vi "Send.vi"(8 "error in (no error)":errorcluster, 10 "Message":refnum<class "BaseMessage.lvclass">, 11 "MultiReader in":refnum<class "MultiReader.lvclass">) -> (0 "error out":errorcluster, 2 "Sent Message":refnum<class "BaseMessage.lvclass">, 3 "MultiReader out":refnum<class "MultiReader.lvclass">)   [LabVIEW 2018, in "MultiReader.lvclass"]
doc: "Send a message to the remote destination"
uses:
  MultiReader.lvclass
  Message/BaseMessage/BaseMessage.lvclass
  MultiReader.lvclass/MultiReader.ctl
  BaseReader/BaseReader.lvclass
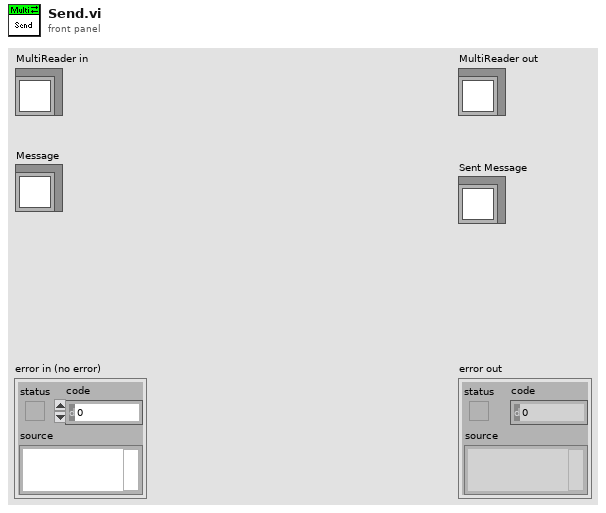
[diagram p1: front panel]
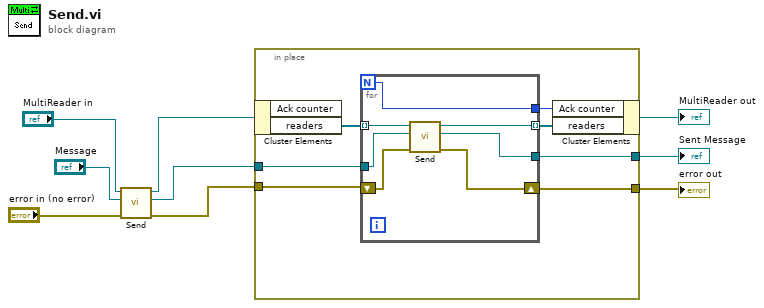
[diagram p0: block diagram]
diagram:
  n1 = call-parent "Send.vi"("error in (no error)"="error in (no error)", "Message"="Message", "BaseReader in"="MultiReader in") -> ("error out"=w4:errorcluster, "Sent Message"=w2:refnum<class "BaseMessage.lvclass">, "BaseReader out"=w6:refnum<class "MultiReader.lvclass">)  [unwired: 6 in]
  n2 = in-place {
    in-place-border: w4 -> [w14]
    in-place-border: [w13] -> w3
    in-place-border: w2 -> [w12]
    in-place-border: [w11] -> w1
    n3 = in-place-cluster #1(w6) -> ("readers"=w16:refnum<class "BaseReader.lvclass">[])  [unwired: 1 out]
    n4 = for {
      N -> [w17]
      tunnel: w16 -> [w23] mode=indexing
      tunnel: [w22] -> w15 mode=indexing
      shift-right: [w19] -> w13
      shift-left: w14 -> [w20]
      tunnel: w12 -> [w21]
      tunnel: [w18] -> w11
      tunnel: [w17] -> w10
      n5 = call-dynamic "Send.vi"("error in (no error)"=w20, "Message"=w21, "BaseReader in"=w23) -> ("error out"=w19:errorcluster, "Sent Message"=w18:refnum<class "BaseMessage.lvclass">, "BaseReader out"=w22:refnum<class "BaseReader.lvclass">)  [unwired: 6 in]
    }
    n6 = in-place-cluster #1("Ack counter"=w10, "readers"=w15) -> (→"MultiReader out":refnum<class "MultiReader.lvclass">)
  }
  "error out" <- w3
  "Sent Message" <- w1
